vi "Controller LNLS Control PS Communication Loop.vi"(7 "Sync Objects":T1, 8 "error in (no error)":errorcluster, 11 "FOFB Configuration":T4={"FOFB Parameters"={"Network"={"FOFB Controller IP"="10.0.18.132", "LNLS Control Network IP"="10.0.18.132", "LNLS Control Network Power Supplies TCP Port"=4001, "LNLS Control Network FOFB Configuration TCP Port"=4002, "LNLS Control Network BPMs TCP Port"=4003, "Monitoring Data TCP Port"=3601, "Fast Archiver TCP Port"=3603, "Fast Command TCP Port"=3604, "TCP Listening Timeout"=-1}, "Fast Acquisition"={"Sampling Period"=320, "Data Buffer Size"=100, "Monitoring Period"=400000}, "Acquisition Network"=[{"Chassis Name"="BPM-Chassis01", "Variables"=[{"Variable Name"="AMP02AH", "Matrix Order"=2, "Plane"=enum."H", "On Correction"=TRUE}, {"Variable Name"="AMP02AV", "Matrix Order"=27, "Plane"=enum."V", "On Correction"=TRUE}, {"Variable Name"="AMP02BH", "Matrix Order"=3, "Plane"=enum."H", "On Correction"=TRUE}, {"Variable Name"="AMP02BV", "Matrix Order"=28, "Plane"=enum."V", "On Correction"=TRUE}, {"Variable Name"="AMP03AH", "Matrix Order"=4, "Plane"=enum."H", "On Correction"=TRUE}, {"Variable Name"="AMP03AV", "Matrix Order"=29, "Plane"=enum."V", "On Correction"=TRUE}, {"Variable Name"="AMP03BH", "Matrix Order"=5, "Plane"=enum."H", "On Correction"=TRUE}, {"Variable Name"="AMP03BV", "Matrix Order"=30, "Plane"=enum."V", "On Correction"=TRUE}, {"Variable Name"="AMP03CH", "Matrix Order"=6, "Plane"=enum."H", "On Correction"=FALSE}, {"Variable Name"="AMP03CV", "Matrix Order"=31, "Plane"=enum."V", "On Correction"=FALSE}]}, {"Chassis Name"="BPM-Chassis02", "Variables"=[{"Variable Name"="AMP04AH", "Matrix Order"=7, "Plane"=enum."H", "On Correction"=TRUE}, {"Variable Name"="AMP04AV", "Matrix Order"=32, "Plane"=enum."V", "On Correction"=TRUE}, {"Variable Name"="AMP04BH", "Matrix Order"=8, "Plane"=enum."H", "On Correction"=TRUE}, {"Variable Name"="AMP04BV", "Matrix Order"=33, "Plane"=enum."V", "On Correction"=TRUE}, {"Variable Name"="AMP05AH", "Matrix Order"=9, "Plane"=enum."H", "On Correction"=TRUE}, {"Variable Name"="AMP05AV", "Matrix Order"=34, "Plane"=enum."V", "On Correction"=TRUE}, {"Variable Name"="AMP05BH", "Matrix Order"=10, "Plane"=enum."H", "On Correction"=TRUE}, {"Variable Name"="AMP05BV", "Matrix Order"=35, "Plane"=enum."V", "On Correction"=TRUE}]}, {"Chassis Name"="BPM-Chassis03", "Variables"=[{"Variable Name"="AMP06AH", "Matrix Order"=11, "Plane"=enum."H", "On Correction"=TRUE}, {"Variable Name"="AMP06AV", "Matrix Order"=36, "Plane"=enum."V", "On Correction"=TRUE}, {"Variable Name"="AMP06BH", "Matrix Order"=12, "Plane"=enum."H", "On Correction"=TRUE}, {"Variable Name"="AMP06BV", "Matrix Order"=37, "Plane"=enum."V", "On Correction"=TRUE}, {"Variable Name"="AMP07AH", "Matrix Order"=13, "Plane"=enum."H", "On Correction"=TRUE}, {"Variable Name"="AMP07AV", "Matrix Order"=38, "Plane"=enum."V", "On Correction"=TRUE}, {"Variable Name"="AMP07BH", "Matrix Order"=14, "Plane"=enum."H", "On Correction"=TRUE}, {"Variable Name"="AMP07BV", "Matrix Order"=39, "Plane"=enum."V", "On Correction"=TRUE}]}, {"Chassis Name"="BPM-Chassis04", "Variables"=[{"Variable Name"="AMP08AH", "Matrix Order"=15, "Plane"=enum."H", "On Correction"=TRUE}, {"Variable Name"="AMP08AV", "Matrix Order"=40, "Plane"=enum."V", "On Correction"=TRUE}, {"Variable Name"="AMP08BH", "Matrix Order"=16, "Plane"=enum."H", "On Correction"=TRUE}, {"Variable Name"="AMP08BV", "Matrix Order"=41, "Plane"=enum."V", "On Correction"=TRUE}, {"Variable Name"="AMP09AH", "Matrix Order"=17, "Plane"=enum."H", "On Correction"=TRUE}, {"Variable Name"="AMP09AV", "Matrix Order"=42, "Plane"=enum."V", "On Correction"=TRUE}, {"Variable Name"="AMP09BH", "Matrix Order"=18, "Plane"=enum."H", "On Correction"=TRUE}, {"Variable Name"="AMP09BV", "Matrix Order"=43, "Plane"=enum."V", "On Correction"=TRUE}]}, {"Chassis Name"="BPM-Chassis05", "Variables"=[{"Variable Name"="AMP10AH", "Matrix Order"=19, "Plane"=enum."H", "On Correction"=TRUE}, {"Variable Name"="AMP10AV", "Matrix Order"=44, "Plane"=enum."V", "On Correction"=TRUE}, {"Variable Name"="AMP10BH", "Matrix Order"=20, "Plane"=enum."H", "On Correction"=TRUE}, {"Variable Name"="AMP10BV", "Matrix Order"=45, "Plane"=enum."V", "On Correction"=TRUE}, {"Variable Name"="AMU11AH", "Matrix Order"=21, "Plane"=enum."H", "On Correction"=TRUE}, {"Variable Name"="AMU11AV", "Matrix Order"=46, "Plane"=enum."V", "On Correction"=TRUE}, {"Variable Name"="AMU11BH", "Matrix Order"=22, "Plane"=enum."H", "On Correction"=TRUE}, {"Variable Name"="AMU11BV", "Matrix Order"=47, "Plane"=enum."V", "On Correction"=TRUE}]}, {"Chassis Name"="BPM-Chassis06", "Variables"=[{"Variable Name"="AMP12AH", "Matrix Order"=23, "Plane"=enum."H", "On Correction"=TRUE}, {"Variable Name"="AMP12AV", "Matrix Order"=48, "Plane"=enum."V", "On Correction"=TRUE}, {"Variable Name"="AMP12BH", "Matrix Order"=24, "Plane"=enum."H", "On Correction"=TRUE}, {"Variable Name"="AMP12BV", "Matrix Order"=49, "Plane"=enum."V", "On Correction"=TRUE}, {"Variable Name"="AMP01AH", "Matrix Order"=25, "Plane"=enum."H", "On Correction"=TRUE}, {"Variable Name"="AMP01AV", "Matrix Order"=50, "Plane"=enum."V", "On Correction"=TRUE}, {"Variable Name"="AMP01BH", "Matrix Order"=1, "Plane"=enum."H", "On Correction"=TRUE}, {"Variable Name"="AMP01BV", "Matrix Order"=26, "Plane"=enum."V", "On Correction"=TRUE}]}], "Actuation Network"=[{"Chassis Name"="PS-RA01B", "Variables"=[{"Variable Name"="ACH01B", "Matrix Order"=1, "Plane"=enum."H", "On Correction"=TRUE}, {"Variable Name"="ACV01B", "Matrix Order"=19, "Plane"=enum."V", "On Correction"=TRUE}, {"Variable Name"="ACH03A", "Matrix Order"=3, "Plane"=enum."H", "On Correction"=TRUE}, {"Variable Name"="ACV03A", "Matrix Order"=22, "Plane"=enum."V", "On Correction"=TRUE}, {"Variable Name"="ALV02A", "Matrix Order"=20, "Plane"=enum."V", "On Correction"=TRUE}, {"Variable Name"="ALV02B", "Matrix Order"=21, "Plane"=enum."V", "On Correction"=TRUE}, {"Variable Name"="ACH02", "Matrix Order"=2, "Plane"=enum."H", "On Correction"=TRUE}]}, {"Chassis Name"="PS-RA02B", "Variables"=[{"Variable Name"="ACH03B", "Matrix Order"=4, "Plane"=enum."H", "On Correction"=TRUE}, {"Variable Name"="ACV03B", "Matrix Order"=23, "Plane"=enum."V", "On Correction"=TRUE}, {"Variable Name"="ACH05A", "Matrix Order"=6, "Plane"=enum."H", "On Correction"=TRUE}, {"Variable Name"="ACV05A", "Matrix Order"=26, "Plane"=enum."V", "On Correction"=TRUE}, {"Variable Name"="ALV04A", "Matrix Order"=24, "Plane"=enum."V", "On Correction"=TRUE}, {"Variable Name"="ALV04B", "Matrix Order"=25, "Plane"=enum."V", "On Correction"=TRUE}, {"Variable Name"="ACH04", "Matrix Order"=5, "Plane"=enum."H", "On Correction"=TRUE}]}, {"Chassis Name"="PS-RA03B", "Variables"=[{"Variable Name"="ACH05B", "Matrix Order"=7, "Plane"=enum."H", "On Correction"=TRUE}, {"Variable Name"="ACV05B", "Matrix Order"=27, "Plane"=enum."V", "On Correction"=TRUE}, {"Variable Name"="ACH07A", "Matrix Order"=9, "Plane"=enum."H", "On Correction"=TRUE}, {"Variable Name"="ACV07A", "Matrix Order"=30, "Plane"=enum."V", "On Correction"=TRUE}, {"Variable Name"="ALV06A", "Matrix Order"=28, "Plane"=enum."V", "On Correction"=TRUE}, {"Variable Name"="ALV06B", "Matrix Order"=29, "Plane"=enum."V", "On Correction"=TRUE}, {"Variable Name"="ACH06", "Matrix Order"=8, "Plane"=enum."H", "On Correction"=TRUE}]}, {"Chassis Name"="PS-RA04B", "Variables"=[{"Variable Name"="ACH07B", "Matrix Order"=10, "Plane"=enum."H", "On Correction"=TRUE}, {"Variable Name"="ACV07B", "Matrix Order"=31, "Plane"=enum."V", "On Correction"=TRUE}, {"Variable Name"="ACH09A", "Matrix Order"=12, "Plane"=enum."H", "On Correction"=TRUE}, {"Variable Name"="ACV09A", "Matrix Order"=34, "Plane"=enum."V", "On Correction"=TRUE}, {"Variable Name"="ALV08A", "Matrix Order"=32, "Plane"=enum."V", "On Correction"=TRUE}, {"Variable Name"="ALV08B", "Matrix Order"=33, "Plane"=enum."V", "On Correction"=TRUE}, {"Variable Name"="ACH08", "Matrix Order"=11, "Plane"=enum."H", "On Correction"=TRUE}]}, {"Chassis Name"="PS-RA05B", "Variables"=[{"Variable Name"="ACH09B", "Matrix Order"=13, "Plane"=enum."H", "On Correction"=TRUE}, {"Variable Name"="ACV09B", "Matrix Order"=35, "Plane"=enum."V", "On Correction"=TRUE}, {"Variable Name"="ACH11A", "Matrix Order"=15, "Plane"=enum."H", "On Correction"=TRUE}, {"Variable Name"="ACV11A", "Matrix Order"=38, "Plane"=enum."V", "On Correction"=TRUE}, {"Variable Name"="ALV10A", "Matrix Order"=36, "Plane"=enum."V", "On Correction"=TRUE}, {"Variable Name"="ALV10B", "Matrix Order"=37, "Plane"=enum."V", "On Correction"=TRUE}, {"Variable Name"="ACH10", "Matrix Order"=14, "Plane"=enum."H", "On Correction"=TRUE}]}, {"Chassis Name"="PS-RA06B", "Variables"=[{"Variable Name"="ACH11B", "Matrix Order"=16, "Plane"=enum."H", "On Correction"=TRUE}, {"Variable Name"="ACV11B", "Matrix Order"=39, "Plane"=enum."V", "On Correction"=TRUE}, {"Variable Name"="ACH01A", "Matrix Order"=18, "Plane"=enum."H", "On Correction"=TRUE}, {"Variable Name"="ACV01A", "Matrix Order"=42, "Plane"=enum."V", "On Correction"=TRUE}, {"Variable Name"="ALV12A", "Matrix Order"=40, "Plane"=enum."V", "On Correction"=TRUE}, {"Variable Name"="ALV12B", "Matrix Order"=41, "Plane"=enum."V", "On Correction"=TRUE}, {"Variable Name"="ACH12", "Matrix Order"=17, "Plane"=enum."H", "On Correction"=TRUE}]}]}, "Number of Acquisition Chassis"=6, "Number of Actuation Chassis"=6, "Number of BPM Readings"=50, "BPM Reading Names"=["AMP01BH", "AMP02AH", "AMP02BH", "AMP03AH", "AMP03BH", "AMP03CH", "AMP04AH", "AMP04BH", "AMP05AH", "AMP05BH", "AMP06AH", "AMP06BH", "AMP07AH", "AMP07BH", "AMP08AH", "AMP08BH", "AMP09AH", "AMP09BH", "AMP10AH", "AMP10BH", "AMU11AH", "AMU11BH", "AMP12AH", "AMP12BH", "AMP01AH", "AMP01BV", "AMP02AV", "AMP02BV", "AMP03AV", "AMP03BV", "AMP03CV", "AMP04AV", "AMP04BV", "AMP05AV", "AMP05BV", "AMP06AV", "AMP06BV", "AMP07AV", "AMP07BV", "AMP08AV", "AMP08BV", "AMP09AV", "AMP09BV", "AMP10AV", "AMP10BV", "AMU11AV", "AMU11BV", "AMP12AV", "AMP12BV", "AMP01AV"], "Selected BPM Readings"=[0, 1, 2, 3, 4, 6, 7, 8, 9, 10, 11, 12, 13, 14, 15, 16, 17, 18, 19, 20, 21, 22, 23, 24, 25, 26, 27, 28, 29, 31, 32, 33, 34, 35, 36, 37, 38, 39, 40, 41, 42, 43, 44, 45, 46, 47, 48, 49], "Number of Correctors"=42, "Corrector Names"=["ACH01B", "ACH02", "ACH03A", "ACH03B", "ACH04", "ACH05A", "ACH05B", "ACH06", "ACH07A", "ACH07B", "ACH08", "ACH09A", "ACH09B", "ACH10", "ACH11A", "ACH11B", "ACH12", "ACH01A", "ACV01B", "ALV02A", "ALV02B", "ACV03A", "ACV03B", "ALV04A", "ALV04B", "ACV05A", "ACV05B", "ALV06A", "ALV06B", "ACV07A", "ACV07B", "ALV08A", "ALV08B", "ACV09A", "ACV09B", "ALV10A", "ALV10B", "ACV11A", "ACV11B", "ALV12A", "ALV12B", "ACV01A"], "Selected Correctors"=[0, 1, 2, 3, 4, 5, 6, 7, 8, 9, 10, 11, 12, 13, 14, 15, 16, 17, 18, 19, 20, 21, 22, 23, 24, 25, 26, 27, 28, 29, 30, 31, 32, 33, 34, 35, 36, 37, 38, 39, 40, 41], "Response Matrix"=[[[-1.09330819, 0.83238826, -1.93923182, -0.39618552, -0.98307235, -1.88049663, 1.00296681, -0.19883275, -1.65005616, -0.55712353, 0.68544531, -0.70274756, -0.65496658, 0.05515979, -0.38935, 0.30350319, -0.13918837, -0.00011801, -0.21517587, -0.53815631, 0.44595451, 0.75898104, -0.44725813, -1.09971674, -0.46972415, -0.36841134, -0.07750092, 0.48295386, 0.47744403, 2.130847, 0.4681161, 0.39999255, -0.15570575, 0.89687682, 0.94383742, 1.1290593, -0.75786475, 0.54152616, 0.43217361, 0.98547068, 0.07993329, 0.29159442, 0.45045343, 0.73064824, 0.57741329, 0.86763439, 1.47745915, 1.05383194, 0.75658237, 0.2512502]]], "Reference Orbit"=array50x42[2100 elements], "Correction Matrix"=array1x42x48[2016 elements], "FPGA Filter Sets"=[], "Acquisition Chassis Names"=["PS-RA01B", "PS-RA02B", "PS-RA03B", "PS-RA04B", "PS-RA05B", "PS-RA06B"], "Actuation Chassis Names"=[], "Acquisition Variables"=[{"Variable Name"="ACH01B", "Chassis Name"="PS-RA01B"}, {"Variable Name"="ACH02", "Chassis Name"="PS-RA01B"}, {"Variable Name"="ACH03A", "Chassis Name"="PS-RA01B"}, {"Variable Name"="ACH03B", "Chassis Name"="PS-RA02B"}, {"Variable Name"="ACH04", "Chassis Name"="PS-RA02B"}, {"Variable Name"="ACH05A", "Chassis Name"="PS-RA02B"}, {"Variable Name"="ACH05B", "Chassis Name"="PS-RA03B"}, {"Variable Name"="ACH06", "Chassis Name"="PS-RA03B"}, {"Variable Name"="ACH07A", "Chassis Name"="PS-RA03B"}, {"Variable Name"="ACH07B", "Chassis Name"="PS-RA04B"}, {"Variable Name"="ACH08", "Chassis Name"="PS-RA04B"}, {"Variable Name"="ACH09A", "Chassis Name"="PS-RA04B"}, {"Variable Name"="ACH09B", "Chassis Name"="PS-RA05B"}, {"Variable Name"="ACH10", "Chassis Name"="PS-RA05B"}, {"Variable Name"="ACH11A", "Chassis Name"="PS-RA05B"}, {"Variable Name"="ACH11B", "Chassis Name"="PS-RA06B"}, {"Variable Name"="ACH12", "Chassis Name"="PS-RA06B"}, {"Variable Name"="ACH01A", "Chassis Name"="PS-RA06B"}, {"Variable Name"="ACV01B", "Chassis Name"="PS-RA01B"}, {"Variable Name"="ALV02A", "Chassis Name"="PS-RA01B"}, {"Variable Name"="ALV02B", "Chassis Name"="PS-RA01B"}, {"Variable Name"="ACV03A", "Chassis Name"="PS-RA01B"}, {"Variable Name"="ACV03B", "Chassis Name"="PS-RA02B"}, {"Variable Name"="ALV04A", "Chassis Name"="PS-RA02B"}, {"Variable Name"="ALV04B", "Chassis Name"="PS-RA02B"}, {"Variable Name"="ACV05A", "Chassis Name"="PS-RA02B"}, {"Variable Name"="ACV05B", "Chassis Name"="PS-RA03B"}, {"Variable Name"="ALV06A", "Chassis Name"="PS-RA03B"}, {"Variable Name"="ALV06B", "Chassis Name"="PS-RA03B"}, {"Variable Name"="ACV07A", "Chassis Name"="PS-RA03B"}, {"Variable Name"="ACV07B", "Chassis Name"="PS-RA04B"}, {"Variable Name"="ALV08A", "Chassis Name"="PS-RA04B"}, {"Variable Name"="ALV08B", "Chassis Name"="PS-RA04B"}, {"Variable Name"="ACV09A", "Chassis Name"="PS-RA04B"}, {"Variable Name"="ACV09B", "Chassis Name"="PS-RA05B"}, {"Variable Name"="ALV10A", "Chassis Name"="PS-RA05B"}, {"Variable Name"="ALV10B", "Chassis Name"="PS-RA05B"}, {"Variable Name"="ACV11A", "Chassis Name"="PS-RA05B"}, {"Variable Name"="ACV11B", "Chassis Name"="PS-RA06B"}, {"Variable Name"="ALV12A", "Chassis Name"="PS-RA06B"}, {"Variable Name"="ALV12B", "Chassis Name"="PS-RA06B"}, {"Variable Name"="ACV01A", "Chassis Name"="PS-RA06B"}], "Actuation Variables"=[{"Variable Name"="", "Chassis Name"=""}, {"Variable Name"="", "Chassis Name"=""}, {"Variable Name"="", "Chassis Name"=""}, {"Variable Name"="", "Chassis Name"=""}, {"Variable Name"="", "Chassis Name"=""}, {"Variable Name"="", "Chassis Name"=""}], "PS Matrix Mapping"=[], "Inverse PS Matrix Mapping"=[], "BPM Matrix Mapping"=[], "Inverse BPM Matrix Mapping"=[[0, 0, 0, 0, 0, 0, 16843008, 16843009, 16843009, 16843009, 16843009, 16843009, 257, 0, 516538096, 516549112, 95143185, 0, 0, 516547907, 33975304, 49, 516550840, 0, 0, 516513040, 2, 0, 0, 0, 0, 0, 516539392, 516544576, 95143185, 0, 0, 516553163, 33975304, 49, 516550840, 0, 0, 516513112, 2, 0, 0, 0, 0, 0]], "BPM Planes"=[enum."H", enum."H", enum."H", enum."H", enum."H", enum."H", enum."H", enum."H", enum."H", enum."H", enum."H", enum."H", enum."H", enum."H", enum."H", enum."H", enum."H", enum."H", enum."V", enum."V", enum."V", enum."V", enum."V", enum."V", enum."V", enum."V", enum."V", enum."V", enum."V", enum."V", enum."V", enum."V", enum."V", enum."V", enum."V", enum."V", enum."V", enum."V", enum."V", enum."V", enum."V", enum."V"], "Corrector Planes"=[]}) -> (0 "error out":errorcluster)   [LabVIEW 2011, in "Controller VIs.lvlib"]
uses:
  Controller VIs.lvlib
  Types Definitions/Type FOFB Configuration.ctl
  Types Definitions/Type FOFB Parameters.ctl
  Types Definitions/Type Network Configuration.ctl
  Types Definitions/Type FA Configuration.ctl
  Types Definitions/Type Acquisition Network Configuration.ctl
  Types Definitions/Type Actuation Network Configuration.ctl
  Types Definitions/Type Synchronization Objects.ctl
  Types Definitions/Type Blocking Synchronization Objects.ctl
  Types Definitions/Type Monitoring Data.ctl
  Types Definitions/Type Operation Mode State.ctl
  Types Definitions/Type Diagnostics Data.ctl
  Types Definitions/Type CPU Loads Array.ctl
  Types Definitions/Type CPU Loads.ctl
  Types Definitions/Type Non-blocking Synchronization Objects.ctl
  Types Definitions/Type FOFB Variables.ctl
  Types Definitions/Type Actuation State.ctl
  Types Definitions/Type TCP State.ctl
  <vilib>/Platform/TimedLoop/XDataNode/timing_clust.ctl
  <vilib>/Platform/TimedLoop/XDataNode/nitl_modes.ctl
  <vilib>/Platform/TimedLoop/XDataNode/wakeup.ctl
  Controller Global Variables/Monitoring Data.vi
  LNLS Control VIs/LNLS Control Saturation minus10 10.vi
  <vilib>/Platform/TimedLoop/XDataNode/XDataNode.xnode
  LNLS Control VIs.lvlib
  Common VIs.lvlib
  Misc VIs.lvlib
  Controller Global Variables.lvlib
  <vilib>/Platform/TimedLoop/XDataNode/XDNodeRunTimeDep.lvlib
  Type Definitions.lvlib
panel:
  in  "send":bool
  in  "PS Status (On correction?)":bool[](array[boolean])=[TRUE, TRUE, TRUE, TRUE, TRUE, TRUE, TRUE, TRUE, TRUE, TRUE, TRUE, TRUE, TRUE, TRUE, TRUE, TRUE, TRUE, TRUE, TRUE, TRUE, TRUE, TRUE, TRUE, TRUE, TRUE, TRUE, TRUE, TRUE, TRUE, TRUE, TRUE, TRUE, TRUE, TRUE, TRUE, TRUE, TRUE, TRUE, TRUE, TRUE, TRUE, TRUE]
  in  "PS Status (ON/OFF)":bool[](array[boolean])=[TRUE, TRUE, TRUE, TRUE, TRUE, TRUE, TRUE, TRUE, TRUE, TRUE, TRUE, TRUE, TRUE, TRUE, TRUE, TRUE, TRUE, TRUE, TRUE, TRUE, TRUE, TRUE, TRUE, TRUE, TRUE, TRUE, TRUE, TRUE, TRUE, TRUE, TRUE, TRUE, TRUE, TRUE, TRUE, TRUE, TRUE, TRUE, TRUE, TRUE, TRUE, TRUE]
  in  "PS Setpoints":dbl[](array[numeric])=[0.0, 0.0, 0.0, 0.0, 0.0, 0.0, 0.0, 0.0, 0.0, 0.0, 0.0, 0.0, 0.0, 0.0, 0.0, 0.0, 0.0, 0.0, 0.0, 0.0, 0.0, 0.0, 0.0, 0.0, 0.0, 0.0, 0.0, 0.0, 0.0, 0.0, 0.0, 0.0, 0.0, 0.0, 0.0, 0.0, 0.0, 0.0, 0.0, 0.0, 0.0, 0.0]
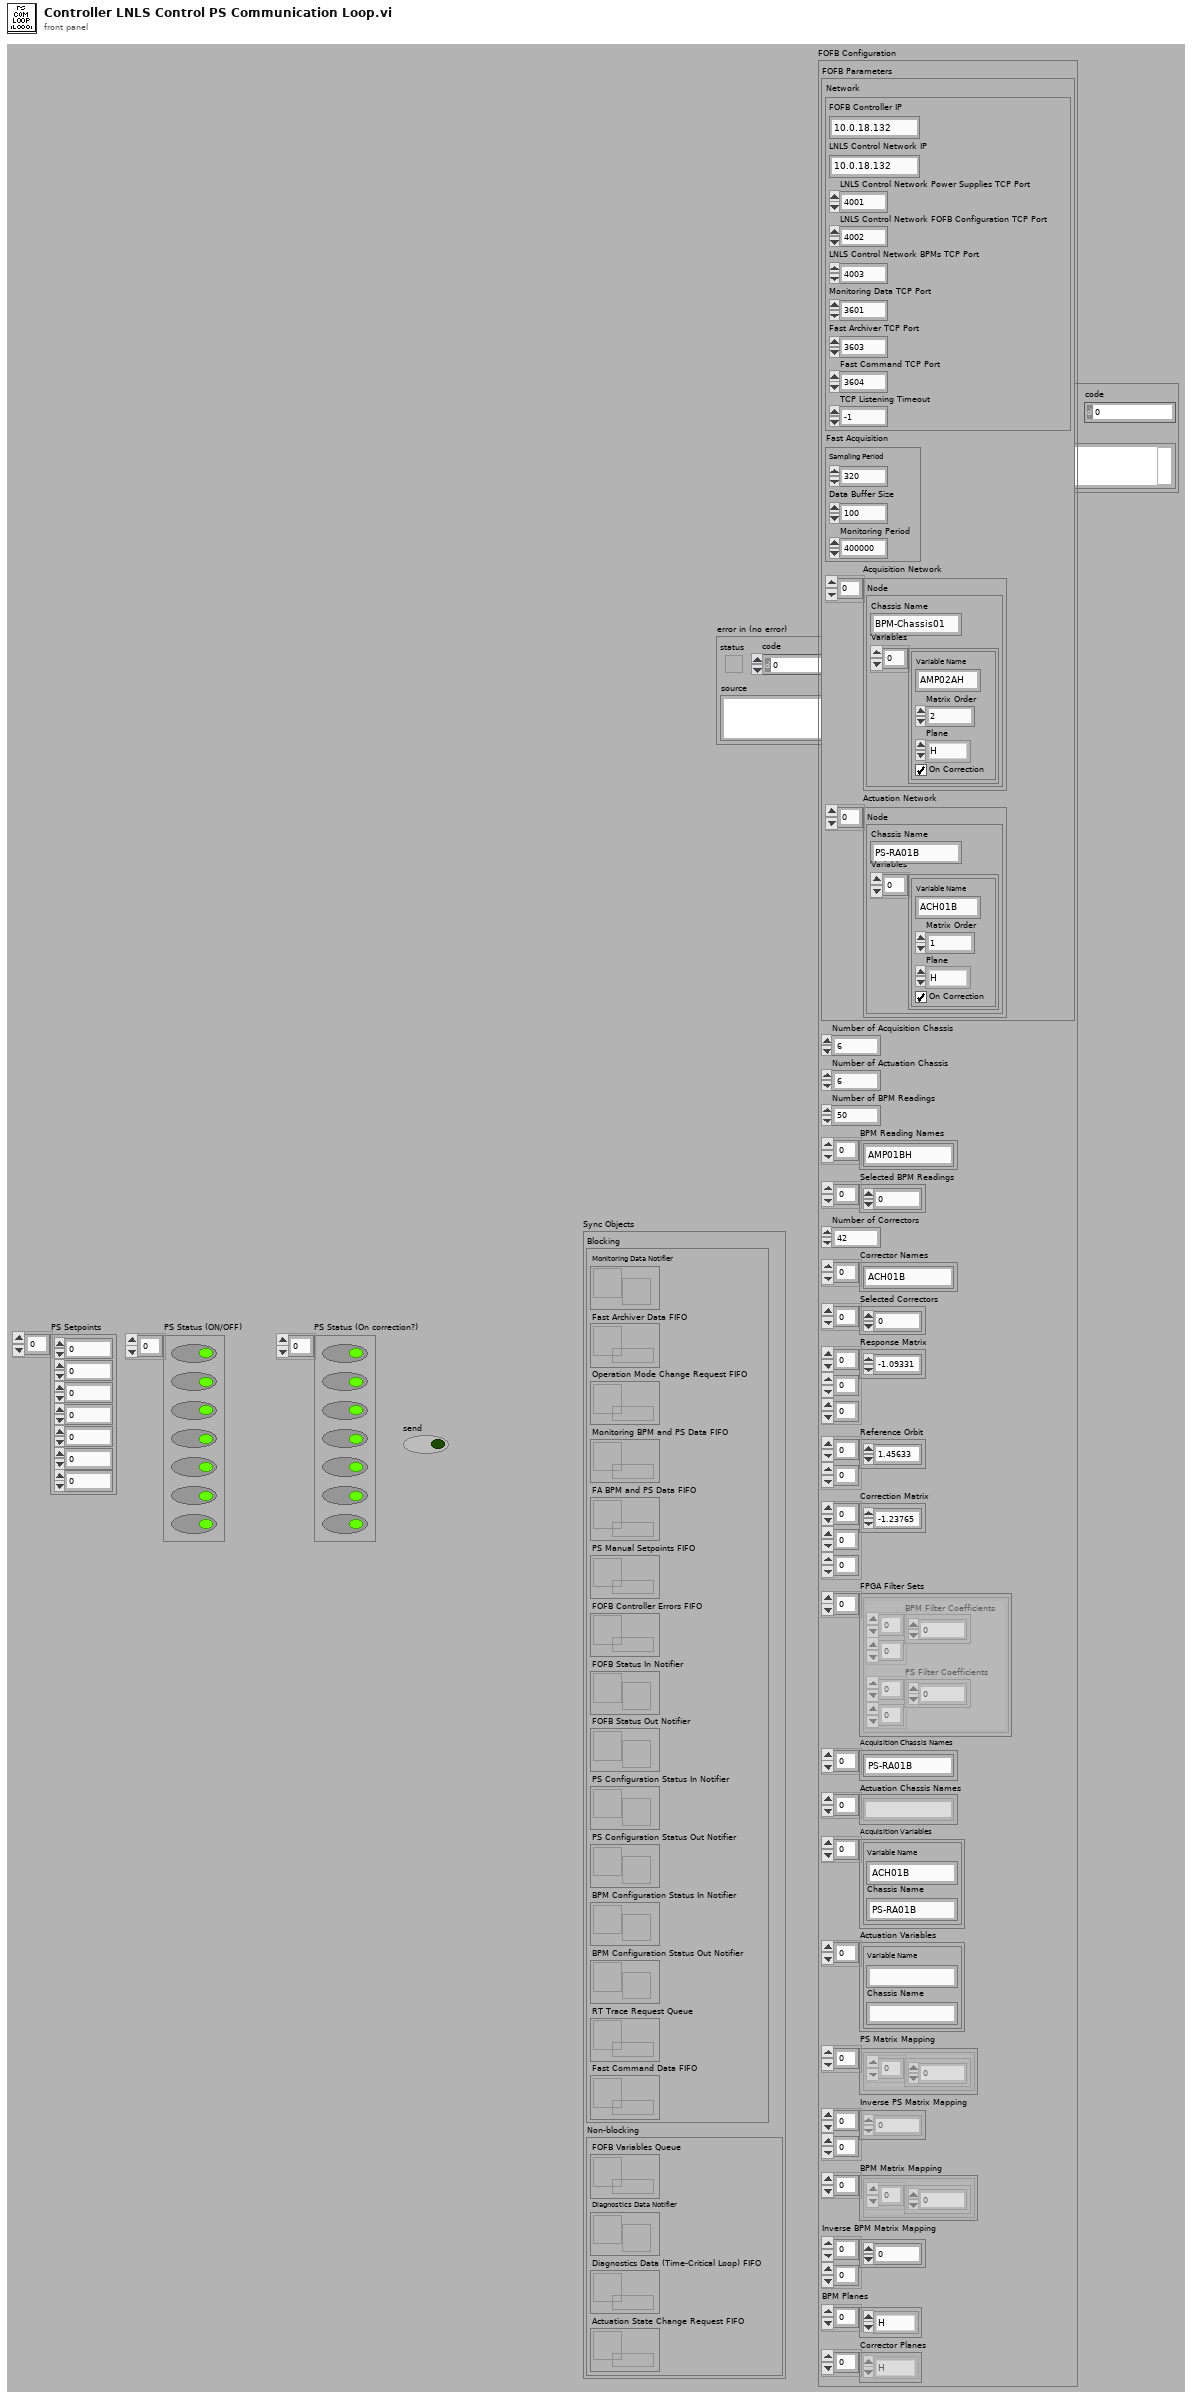
[diagram p1: front panel]
types:
  T1 = typedef "Type Definitions.lvlib/Type Synchronization Objects.ctl" = cluster{"Blocking":T2, "Non-blocking":T3}
  T2 = typedef "Type Definitions.lvlib/Type Blocking Synchronization Objects.ctl" = cluster{"Monitoring Data Notifier":refnum<notifier>, "Fast Archiver Data FIFO":refnum<queue>, "Operation Mode Change Request FIFO":refnum<k33>, "Monitoring BPM and PS Data FIFO":refnum<k33>, "FA BPM and PS Data FIFO":refnum<k33>, "PS Manual Setpoints FIFO":refnum<k33>, "FOFB Controller Errors FIFO ":refnum<k33>, "FOFB Status In Notifier":refnum<notifier>, "FOFB Status Out Notifier":refnum<notifier>, "PS Configuration Status In Notifier":refnum<notifier>, "PS Configuration Status Out Notifier":refnum<notifier>, "BPM Configuration Status In Notifier":refnum<notifier>, "BPM Configuration Status Out Notifier":refnum<notifier>, "RT Trace Request Queue":refnum<queue>, "Fast Command Data FIFO":refnum<k33>}
  T3 = typedef "Type Definitions.lvlib/Type Non-blocking Synchronization Objects.ctl" = cluster{"FOFB Variables Queue":refnum<queue>, "Diagnostics Data Notifier":refnum<notifier>, "Diagnostics Data (Time-Critical Loop) FIFO":refnum<k33>, "Actuation State Change Request FIFO":refnum<k33>}
  T4 = typedef "Type Definitions.lvlib/Type FOFB Configuration.ctl" = cluster{"FOFB Parameters":T5, "Number of Acquisition Chassis":i32, "Number of Actuation Chassis":i32, "Number of BPM Readings":i32, "BPM Reading Names":string[], "Selected BPM Readings":u32[], "Number of Correctors":i32, "Corrector Names":string[], "Selected Correctors":u32[], "Response Matrix":dbl[][][], "Reference Orbit":dbl[][], "Correction Matrix":dbl[][][], "FPGA Filter Sets":cluster{"BPM Filter Coefficients":dbl[][], "PS Filter Coefficients":dbl[][]}[], "Acquisition Chassis Names":string[], "Actuation Chassis Names":string[], "Acquisition Variables":cluster{"Variable Name":string, "Chassis Name":string}[], "Actuation Variables":cluster{"Variable Name":string, "Chassis Name":string}[], "PS Matrix Mapping":cluster{u32[]}[], "Inverse PS Matrix Mapping":u32[][], "BPM Matrix Mapping":cluster{u32[]}[], "Inverse BPM Matrix Mapping":u32[][], "BPM Planes":enum8{"H", "V"}[], "Corrector Planes":enum8{"H", "V"}[]}
  T5 = typedef "Type Definitions.lvlib/Type FOFB Parameters.ctl" = cluster{"Network":T6, "Fast Acquisition":T7, "Acquisition Network":T8, "Actuation Network":T9}
  T6 = typedef "Type Definitions.lvlib/Type Network Configuration.ctl" = cluster{"FOFB Controller IP":string, "LNLS Control Network IP":string, "LNLS Control Network Power Supplies TCP Port":u16, "LNLS Control Network FOFB Configuration TCP Port":u16, "LNLS Control Network BPMs TCP Port":u16, "Monitoring Data TCP Port":u16, "Fast Archiver TCP Port":u16, "Fast Command TCP Port":u16, "TCP Listening Timeout":i32}
  T7 = typedef "Type Definitions.lvlib/Type FA Configuration.ctl" = cluster{"Sampling Period":u32, "Data Buffer Size":u32, "Monitoring Period":u32}
  T8 = typedef "Type Definitions.lvlib/Type Acquisition Network Configuration.ctl" = cluster{"Chassis Name":string, "Variables":cluster{"Variable Name":string, "Matrix Order":u32, "Plane":enum8{"H", "V"}, "On Correction":bool}[]}[]
  T9 = typedef "Type Definitions.lvlib/Type Actuation Network Configuration.ctl" = cluster{"Chassis Name":string, "Variables":cluster{"Variable Name":string, "Matrix Order":u32, "Plane":enum8{"H", "V"}, "On Correction":bool}[]}[]
  T10 = typedef "Type Definitions.lvlib/Type TCP State.ctl" = enum16{"Idle", "Wait Connection", "Read Data", "Process Data", "Write Data", "Close Connection"}
  T11 = typedef "XDNodeRunTimeDep.lvlib/timing_clust.ctl" = cluster{"Expected End [f-1]":u64, "Actual End [f-1]":u64, "Finished Late? [f-1]":bool, "Expected End [i-1]":u64, "Actual End [i-1]":u64, "Finished Late? [i-1]":bool, "Expected Start [i]":u64, "Actual Start [i]":u64, "Expected Start [f]":u64, "Actual Start [f]":u64, "Source Name":string, "Structure Name":string, "Period":i64, "Deadline":i64, "Offset":i64, "Start":i64, "Priority":i32, "Timeout":i32, "Mode":T12, "Wakeup Reason":T13, "Error":errorcluster, "Source Type":string, "Secondary Source Type":string, "Global End Time":u64, "Global Start Time":u64, "Frame Duration":u64, "Iteration Duration":u64, "Assigned CPU":i32, "I/O Scan Engine Mode":u32}
  T12 = typedef "XDNodeRunTimeDep.lvlib/nitl_modes.ctl" = enum32{"No Change", "Process missed periods, maintain original phase", "Discard missed periods, maintain original phase", "Process missed periods, ignore original phase", "Discard missed periods, ignore original phase"}
  T13 = typedef "XDNodeRunTimeDep.lvlib/wakeup.ctl" = enum32{"Normal", "Aborted", "Asynchronous wakeup", "Timing source error", "Timed loop error", "Timeout"}
  T14 = typedef "Type Definitions.lvlib/Type Monitoring Data.ctl" = cluster{"Timestamp":timestamp, "BPM Readings":dbl[], "PS Readings":dbl[], "PS FOFB Setpoints":dbl[], "PS Status per Rack":u8[], "PS ON-OFF per Rack":u8[], "Operation Mode":T15, "Diagnostics Data":T16, "Controller Status Table":i32[]}
  T15 = typedef "Type Definitions.lvlib/Type Operation Mode State.ctl" = enum8{"Idle Mode", "Manual Mode", "FOFB Mode"}
  T16 = typedef "Type Definitions.lvlib/Type Diagnostics Data.ctl" = cluster{"Time-Critical Loop Missed Iterations":u32, "Time-Critical Loop Execution Time (usec)":u32, "Available Memory (bytes)":u32, "CPU Loads Array":T17}
  T17 = typedef "Type Definitions.lvlib/Type CPU Loads Array.ctl" = T18[]
  T18 = typedef "Type Definitions.lvlib/Type CPU Loads.ctl" = cluster{"Total (%)":dbl, "Time Critical (%)":dbl, "Timed Structures (%)":dbl, "High (%)":dbl, "Above Normal (%)":dbl, "Normal (%)":dbl, "Background (%)":dbl, "Idle (%)":dbl, "ISR (%)":dbl}
  T19 = typedef "Type Definitions.lvlib/Type LOCON_BIPOLAR_16BITS.ctl" = cluster{"priority":u8, "flags":u8, "analog value":u16, "status":u8}
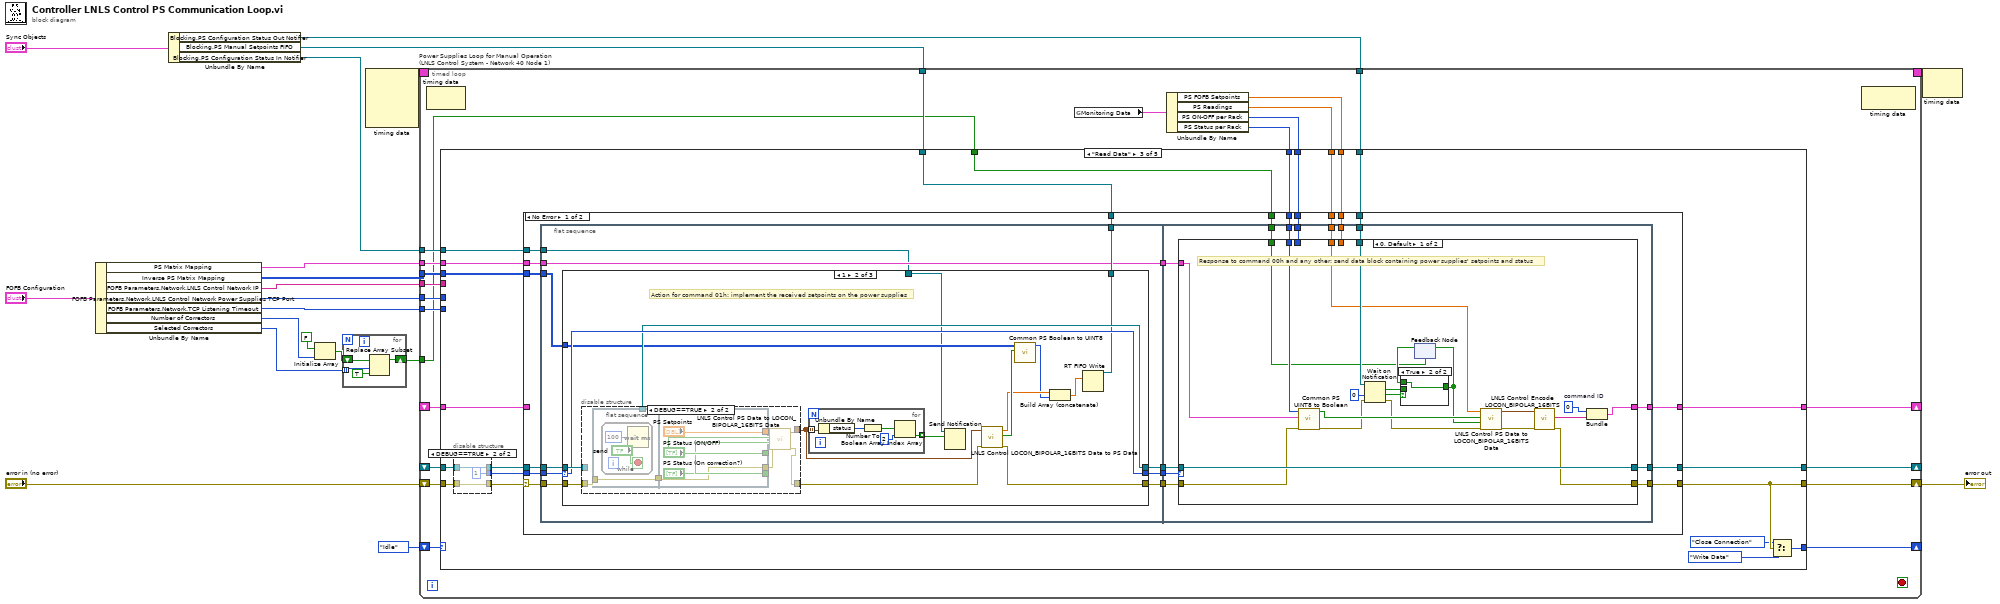
[diagram p0: block diagram]
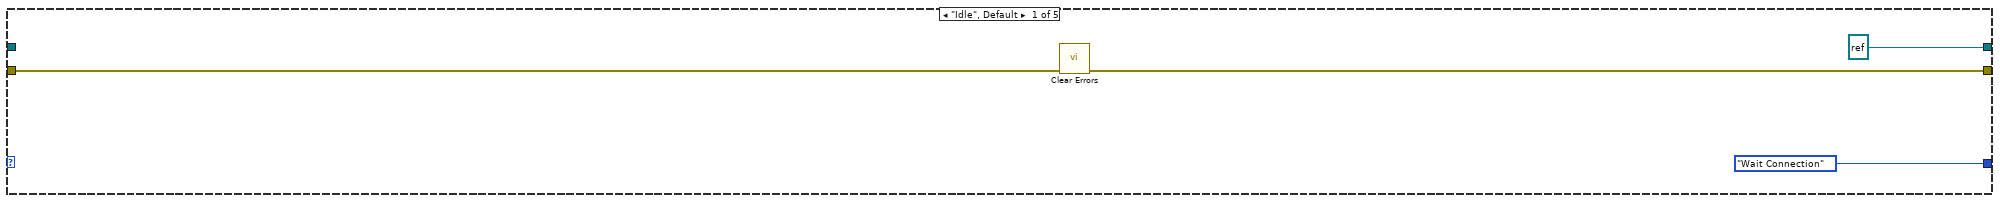
[diagram p2: hidden frame]
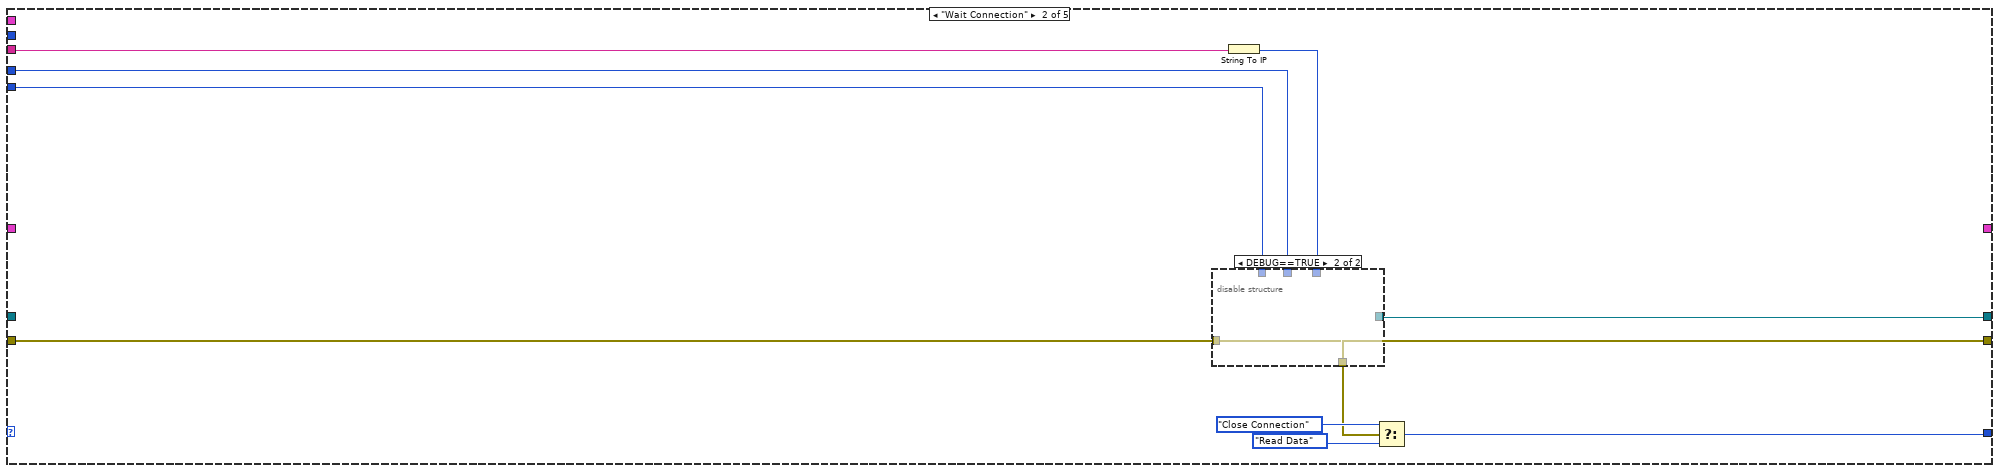
[diagram p3: hidden frame]
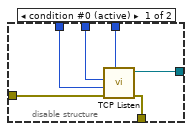
[diagram p4: hidden frame]
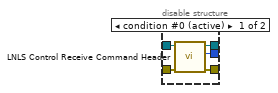
[diagram p5: hidden frame]
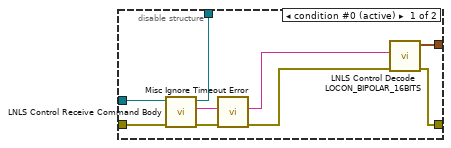
[diagram p7: hidden frame]
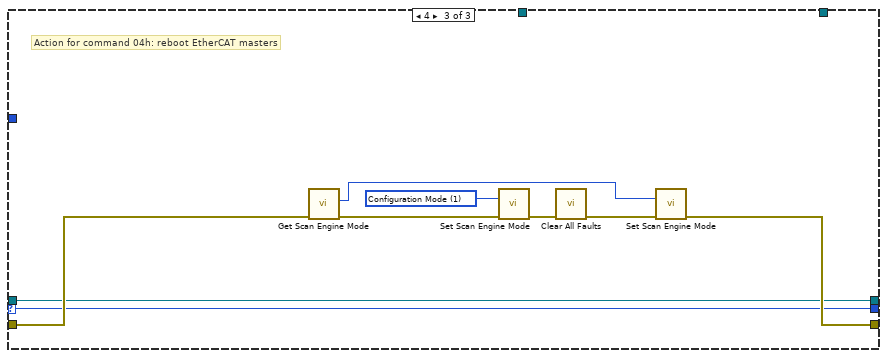
[diagram p8: hidden frame]
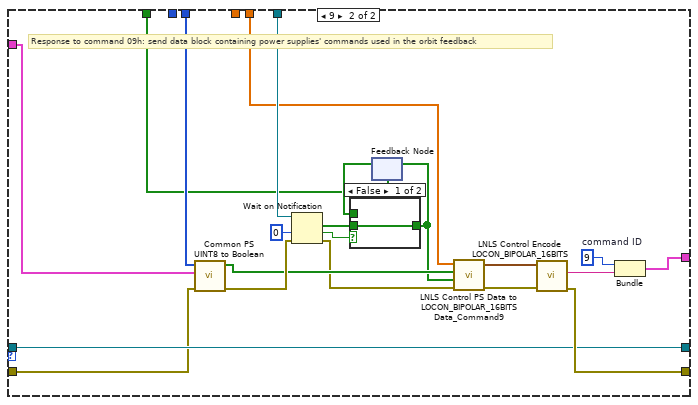
[diagram p10: hidden frame]
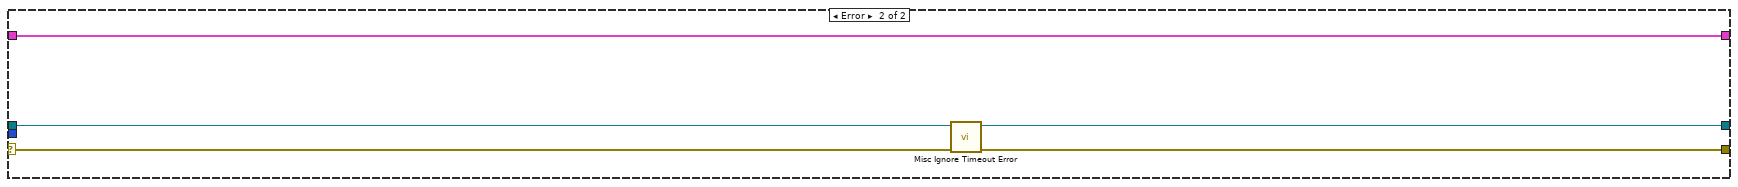
[diagram p12: hidden frame]
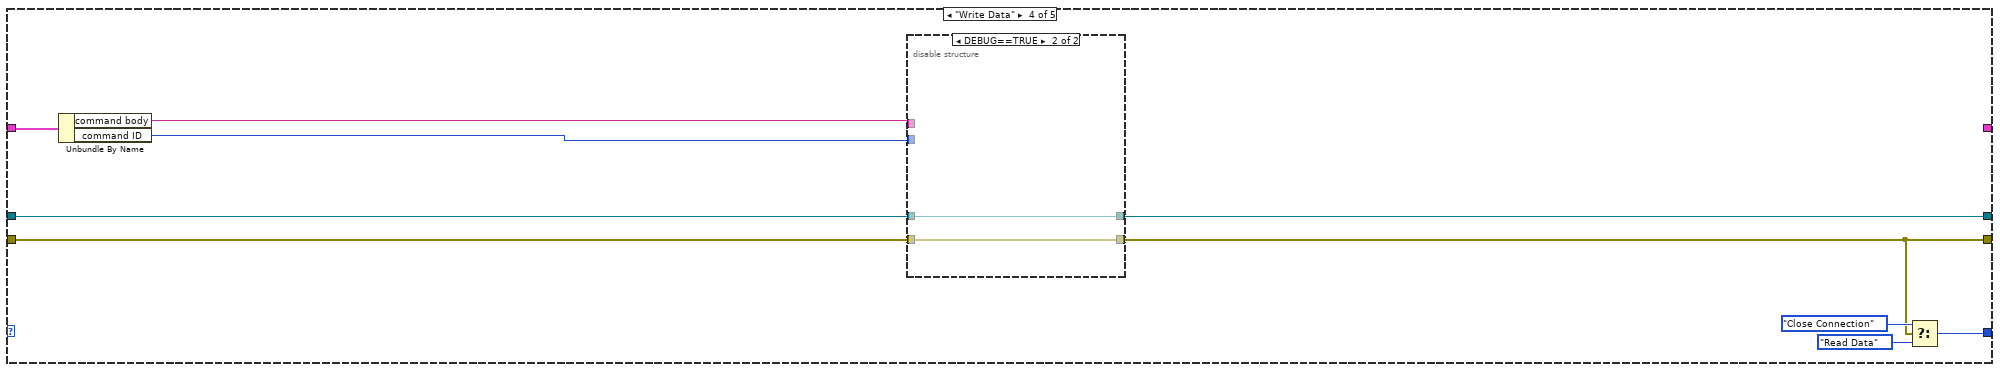
[diagram p13: hidden frame]
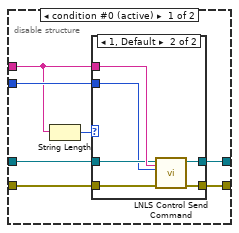
[diagram p14: hidden frame]
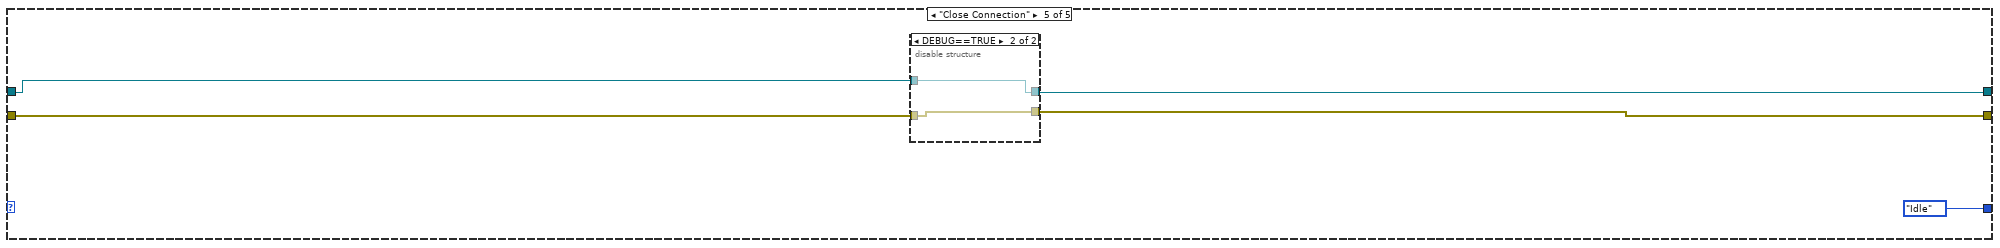
[diagram p16: hidden frame]
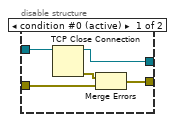
[diagram p17: hidden frame]
diagram:
  n1 = Unbundle By Name("FOFB Configuration") -> ("PS Matrix Mapping"=w13:cluster{u32[]}[], "Inverse PS Matrix Mapping"=w14:u32[][], "FOFB Parameters.Network.LNLS Control Network IP"=w15:string, "FOFB Parameters.Network.LNLS Control Network Power Supplies TCP Port"=w12:u16, "FOFB Parameters.Network.TCP Listening Timeout"=w11:i32, "Number of Correctors"=w5:i32, "Selected Correctors"=w3:u32[])
  n2 = Unbundle By Name("Sync Objects") -> ("Blocking.PS Configuration Status Out Notifier"=w8:refnum<notifier>, "Blocking.PS Manual Setpoints FIFO"=w1:refnum<k33>, "Blocking.PS Configuration Status In Notifier"=w7:refnum<notifier>)
  n3 = Initialize Array(FALSE, w5) -> (w4:bool[])
  n4 = for {
    tunnel: w3 -> [w24] mode=indexing
    shift-right: [w21] -> w2
    shift-left: w4 -> [w23]
    n5 = Replace Array Subset(array=w23, new element=TRUE ("new element/subarray"), index=w24) -> (w21:bool[])
  }
  n6 = node-c288() -> (w10:T11)  [unwired: 4 in]
  n7 = timed-loop "Power Supplies Loop for Manual Operation (LNLS Control System - Network 40 Node 1)" {
    shift-right: [w44] -> _
    shift-left: Type_TCP_State."Idle" ("f") -> [w46]
    shift-right: [w45] -> _
    shift-left: _ -> [w43]
    shift-right: [w25] -> w18
    shift-left: "error in (no error)" -> [w39]
    shift-right: [w41] -> _
    shift-left: _ -> [w40]
    tunnel: w12 -> [w42]
    tunnel: w15 -> [w38]
    tunnel: w14 -> [w37]
    tunnel: w13 -> [w36]
    tunnel: w11 -> [w35]
    tunnel: w1 -> [w31]
    timing: w10 -> [_]
    timing-out: [_] -> w9
    tunnel: w8 -> [w28]
    tunnel: w7 -> [w27]
    tunnel: w2 -> [w26]
    stop <- _ stop-if-true
    n8 = node-c288() -> ()  [unwired: 1 in, 1 out]
    n9 = global read "Monitoring Data.vi" "Monitoring Data"() -> (w32:T14)
    n10 = Unbundle By Name(w32) -> ("PS FOFB Setpoints"=w34:dbl[], "PS Readings"=w33:dbl[], "PS ON-OFF per Rack"=w29:u8[], "PS Status per Rack"=w30:u8[])
    n11 = case shown="\"Read Data\"" w46 {
      tunnel: [refnum<k5> refnum ("connection ID") w59 w91 w251 w278] -> w45
      tunnel: [w50 w54 w89 w250 w275] -> w25
      tunnel: [Type_TCP_State."Wait Connection" w62 w90 w255 Type_TCP_State."Idle"] -> w44
      tunnel: w43 -> [_ _ w87 w253 w279]
      tunnel: w39 -> [w49 w55 w88 w252 w276]
      tunnel: w42 -> [_ w58 _ _ _]
      tunnel: [_ _ w84 _ _] -> w41
      tunnel: w40 -> [_ _ w82 w254 _]
      tunnel: w38 -> [_ w56 _ _ _]
      tunnel: w37 -> [_ _ w80 _ _]
      tunnel: w36 -> [_ _ w79 _ _]
      tunnel: w35 -> [_ w53 _ _ _]
      tunnel: w34 -> [_ _ w70 _ _]
      tunnel: w33 -> [_ _ w71 _ _]
      tunnel: w30 -> [_ _ w78 _ _]
      tunnel: w31 -> [_ _ w77 _ _]
      tunnel: w29 -> [_ _ w76 _ _]
      tunnel: w28 -> [_ _ w75 _ _]
      tunnel: w27 -> [_ _ w73 _ _]
      tunnel: w26 -> [_ _ w72 _ _]
      frame "Idle", Default {
        n12 = call <vilib>:"Clear Errors.vi"("error in (no error)"=w49) -> ("error out"=w50:errorcluster)  [unwired: 6 in]
      }
      frame "Wait Connection" {
        n13 = String To IP(1:w56) -> (0:w57:u32)
        n14 = disable-structure shown="DEBUG==TRUE" {
          disable-tunnel: [w68 _] -> w59
          disable-tunnel: w58 -> [w67 _]
          disable-tunnel: w57 -> [w66 _]
          disable-tunnel: w55 -> [w65 w69]
          disable-tunnel: [w64 w69] -> w54
          disable-tunnel: w53 -> [w63 _]
          frame condition #0 (active) {
            n15 = call <vilib>:"TCP Listen.vi"("net address"=w66, "error in (no error)"=w65, "timeout ms (wait forever: -1)"=w63, "port"=w67) -> ("error out"=w64:errorcluster, "connection ID"=w68:refnum<k5>)  [unwired: 3 in, 3 out]
          }
          frame condition #1 {
          }
        }
        n16 = Select(t=Type_TCP_State."Close Connection", s=w54, f=Type_TCP_State."Read Data") -> (s? t:f=w62:T10)
      }
      frame "Read Data" {
        n17 = disable-structure shown="DEBUG==TRUE" {
          disable-tunnel: w88 -> [w96 w99]
          disable-tunnel: w87 -> [w95 w98]
          disable-tunnel: [w94 w98] -> w86
          disable-tunnel: [w93 w99] -> w83
          disable-tunnel: [w92 u8 1 ("command ID")] -> w74
          frame condition #0 (active) {
            n18 = call "LNLS Control Receive Command Header.vi"("error in (no error)"=w96, "connection ID"=w95) -> ("error out"=w93:errorcluster, "command ID"=w92:u8, "connection ID out"=w94:refnum<k5>)  [unwired: 7 in]
          }
          frame condition #1 {
          }
        }
        n19 = case shown="No Error" w83 {
          selector: w83 -> [w114 w244]
          tunnel: [w119 w247] -> w91
          tunnel: [w118 w245] -> w89
          tunnel: w86 -> [w117 w247]
          tunnel: w74 -> [w116 _]
          tunnel: [w115 w246] -> w84
          tunnel: w82 -> [_ w246]
          tunnel: w80 -> [w110 _]
          tunnel: w79 -> [w108 _]
          tunnel: w70 -> [w107 _]
          tunnel: w71 -> [w106 _]
          tunnel: w78 -> [w105 _]
          tunnel: w77 -> [w104 _]
          tunnel: w76 -> [w103 _]
          tunnel: w75 -> [w102 _]
          tunnel: w73 -> [w101 _]
          tunnel: w72 -> [w100 _]
          frame No Error {
            n20 = flat-sequence {
              tunnel: [w129] -> w113
              tunnel: [w128] -> w112
              tunnel: w117 -> [w127]
              tunnel: w116 -> [w126]
              tunnel: w114 -> [w125]
              tunnel: [w124] -> w111
              tunnel: w110 -> [w123]
              tunnel: [w121] -> w109
              tunnel: w108 -> [w121]
              tunnel: w104 -> [w122]
              tunnel: w101 -> [w120]
              tunnel: [w194] -> w119
              tunnel: w113 -> [w193]
              tunnel: [w197] -> w118
              tunnel: w112 -> [w196]
              tunnel: [w192] -> w115
              tunnel: w111 -> [w195]
              tunnel: w109 -> [w191]
              tunnel: w107 -> [w190]
              tunnel: w106 -> [w189]
              tunnel: w105 -> [w188]
              tunnel: w103 -> [w187]
              tunnel: w102 -> [w186]
              tunnel: w100 -> [w185]
              frame #0 {
                n21 = case shown="1" w126 {
                  selector: w126 -> [w130 w144 w177]
                  tunnel: w125 -> [w132 w146 w184]
                  tunnel: [w132 w145 w183] -> w128
                  tunnel: [w131 w143 w176] -> w129
                  tunnel: w127 -> [w131 w147 w176]
                  tunnel: [w130 w144 w177] -> w124
                  tunnel: w123 -> [_ w142 _]
                  tunnel: w122 -> [_ w140 _]
                  tunnel: w120 -> [_ w135 _]
                  frame 0, Default {
                  }
                  frame 1 {
                    # "Action for command 01h: implement the received setpoints on the power supplies"
                    n22 = disable-structure shown="DEBUG==TRUE" {
                      disable-tunnel: w147 -> [w155 _]
                      disable-tunnel: w146 -> [w154 w159]
                      disable-tunnel: [w153 _] -> w143
                      disable-tunnel: [w149 w163] -> w136
                      disable-tunnel: [w148 w157] -> w134
                      frame condition #0 (active) {
                        n23 = call "LNLS Control Receive Command Body.vi"("error in (no error)"=w154, "connection ID"=w155) -> ("error out"=w150:errorcluster, "command body"=w151:string, "connection ID out"=w153:refnum<k5>)  [unwired: 6 in, 1 out]
                        n24 = call "Misc Ignore Timeout Error.vi"("error in (no error)"=w150) -> ("error out"=w152:errorcluster)  [unwired: 9 in, 1 out]
                        n25 = call "LNLS Control Decode LOCON_BIPOLAR_16BITS.vi"("error in (no error)"=w152, "command body"=w151) -> ("error out"=w148:errorcluster, "LOCON data"=w149:T19[])  [unwired: 6 in]
                      }
                      frame condition #1 {
                        n26 = flat-sequence {
                          tunnel: w159 -> [w164]
                          tunnel: [w164] -> w156
                          tunnel: ["PS Setpoints"] -> w162
                          tunnel: ["PS Status (ON/OFF)"] -> w161
                          tunnel: ["PS Status (On correction?)"] -> w160
                          tunnel: [w167] -> w158
                          tunnel: w156 -> [w167]
                          frame #0 {
                            n27 = while {
                              stop <- "send" stop-if-true
                              n28 = Wait (ms)(milliseconds to wait=u32 100) -> ()  [unwired: 1 out]
                            }
                          }
                          frame #1 {
                          }
                        }
                        n29 = call "LNLS Control PS Data to LOCON_BIPOLAR_16BITS Data.vi"("error in (no error)"=w158, "PS Status (On correction?)"=w160, "PS Status (ON/OFF)"=w161, "PS Readings/Setpoints"=w162) -> ("error out"=w157:errorcluster, "PS Readings/Setpoints LOCON Data"=w163:T19[])  [unwired: 6 in]
                      }
                    }
                    n30 = for {
                      tunnel: w136 -> [w175] mode=indexing
                      tunnel: [w173] -> w133 mode=indexing
                      n31 = Unbundle By Name(w175) -> ("status"=w172:u8)
                      n32 = Number To Boolean Array(number=w172) -> (Boolean array=w171:bool[])
                      n33 = Index Array(array=w171, index=2) -> (element=w173:bool)
                    }
                    n34 = Send Notification(notification=w133, notifier=w135) -> ()  [unwired: 1 in, 2 out]
                    n35 = call "LNLS Control LOCON_BIPOLAR_16BITS Data to PS Data.vi"("error in (no error)"=w134, "PS Setpoints LOCON Data"=w136) -> ("error out"=w145:errorcluster, "PS Status"=w141:bool[], "PS Setpoints"=w139:dbl[])  [unwired: 7 in]
                    n36 = call "Common PS Boolean to UINT8.vi"("PS ON-OFF"=w141, "Inverse PS Matrix Mapping"=w142) -> ("PS ON-OFF (per PS Rack)"=w138:u8[])  [unwired: 8 in, 1 out]
                    n37 = Build Array (concatenate)(w139, w138) -> (w137:dbl[])
                    n38 = RT FIFO Write(0:w140, 1:w137) -> ()  [unwired: 3 in, 4 out]
                  }
                  frame 4 {
                    w182 = 1 items=["Configuration Mode"=1, "Active Mode"=2] ("mode (Active Mode)")
                    # "Action for command 04h: reboot EtherCAT masters"
                    n39 = call <vilib>:"Get Scan Engine Mode.vi"("error in (no error)"=w184) -> ("error out"=w181:errorcluster, "mode"=w178:i32)  [unwired: 9 in]
                    n40 = call <vilib>:"Set Scan Engine Mode.vi"("mode (Active Mode)"=w182, "error in (no error)"=w181) -> ("error out"=w180:errorcluster)  [unwired: 13 in]
                    n41 = call <vilib>:"Clear All Faults.vi"("error in (no error)"=w180) -> ("error out"=w179:errorcluster)  [unwired: 1 in, 9 out]
                    n42 = call <vilib>:"Set Scan Engine Mode.vi"("mode (Active Mode)"=w178, "error in (no error)"=w179) -> ("error out"=w183:errorcluster)  [unwired: 13 in]
                  }
                }
              }
              frame #1 {
                n43 = case shown="0, Default" w195 {
                  tunnel: w196 -> [w213 w236]
                  tunnel: [w214 w239] -> w197
                  tunnel: [w218 w238] -> w194
                  tunnel: w193 -> [w218 w238]
                  tunnel: [w215 w237] -> w192
                  tunnel: w191 -> [w212 w235]
                  tunnel: w190 -> [_ w226]
                  tunnel: w189 -> [w198 _]
                  tunnel: w188 -> [w210 _]
                  tunnel: w187 -> [_ w234]
                  tunnel: w186 -> [w207 w233]
                  tunnel: w185 -> [w199 w227]
                  frame 0, Default {
                    w216 = u8 0  # command ID
                    # "Response to command 00h and any other: send data block containing power supplies' setpoints and status"
                    n44 = call "Common PS UINT8 to Boolean.vi"("error in (no error)"=w213, "PS Matrix Mapping"=w212, "PS Status (per PS Rack)"=w210) -> ("error out"=w206:errorcluster, "PS Status"=w208:bool[])  [unwired: 7 in]
                    n45 = Wait on Notification(notifier=w207, timeout in ms (-1)=0, error in (no error)=w206) -> (notification=w203:bool[], timed out?=w204:bool, error out=w205:errorcluster)  [unwired: 1 in, 1 out]
                    n46 = feedback #1(w199) -> (w200:bool[])
                    n47 = case shown="True" w204 {
                      tunnel: w203 -> [w219 _]
                      tunnel: [w219 w220] -> w201
                      tunnel: w200 -> [_ w220]
                      frame False {
                      }
                      frame True {
                      }
                    }
                    n48 = feedback-in #1(w201) -> ()
                    n49 = call "LNLS Control PS Data to LOCON_BIPOLAR_16BITS Data.vi"("error in (no error)"=w205, "PS Status (On correction?)"=w201, "PS Status (ON/OFF)"=w208, "PS Readings/Setpoints"=w198) -> ("error out"=w217:errorcluster, "PS Readings/Setpoints LOCON Data"=w209:T19[])  [unwired: 6 in]
                    n50 = call "LNLS Control Encode LOCON_BIPOLAR_16BITS.vi"("error in (no error)"=w217, "LOCON Data"=w209) -> ("error out"=w214:errorcluster, "command body"=w211:string)  [unwired: 8 in]
                    n51 = Bundle("command ID"=w216, "command body"=w211) -> (w215:cluster{"command ID":u8, "command body":string})  [unwired: 1 in]
                  }
                  frame 9 {
                    w240 = u8 9  # command ID
                    # "Response to command 09h: send data block containing power supplies' commands used in the orbit feedback"
                    n52 = call "Common PS UINT8 to Boolean.vi"("error in (no error)"=w236, "PS Matrix Mapping"=w235, "PS Status (per PS Rack)"=w234) -> ("error out"=w232:errorcluster, "PS Status"=w225:bool[])  [unwired: 7 in]
                    n53 = Wait on Notification(notifier=w233, timeout in ms (-1)=0, error in (no error)=w232) -> (notification=w229:bool[], timed out?=w228:bool, error out=w223:errorcluster)  [unwired: 1 in, 1 out]
                    n54 = feedback #2(w227) -> (w230:bool[])
                    n55 = case shown="False" w228 {
                      tunnel: w229 -> [w242 _]
                      tunnel: [w242 w243] -> w224
                      tunnel: w230 -> [_ w243]
                      frame False {
                      }
                      frame True {
                      }
                    }
                    n56 = feedback-in #2(w224) -> ()
                    n57 = call "LNLS Control PS Data to LOCON_BIPOLAR_16BITS Data_Command9.vi"("error in (no error)"=w223, "PS Status (On correction?)"=w224, "PS Status (ON/OFF)"=w225, "PS Readings/Setpoints"=w226) -> ("error out"=w221:errorcluster, "PS Readings/Setpoints LOCON Data"=w222:T19[])  [unwired: 6 in]
                    n58 = call "LNLS Control Encode LOCON_BIPOLAR_16BITS.vi"("error in (no error)"=w221, "LOCON Data"=w222) -> ("error out"=w239:errorcluster, "command body"=w241:string)  [unwired: 8 in]
                    n59 = Bundle("command ID"=w240, "command body"=w241) -> (w237:cluster{"command ID":u8, "command body":string})  [unwired: 1 in]
                  }
                }
              }
            }
          }
          frame Error {
            n60 = call "Misc Ignore Timeout Error.vi"("error in (no error)"=w244) -> ("error out"=w245:errorcluster)  [unwired: 9 in, 1 out]
          }
        }
        n61 = Select(t=Type_TCP_State."Close Connection", s=w89, f=Type_TCP_State."Write Data") -> (s? t:f=w90:T10)
      }
      frame "Write Data" {
        n62 = Unbundle By Name(w254) -> ("command body"=w248:string, "command ID"=w249:u8)
        n63 = disable-structure shown="DEBUG==TRUE" {
          disable-tunnel: w253 -> [w264 w273]
          disable-tunnel: w252 -> [w263 w274]
          disable-tunnel: [w262 w273] -> w251
          disable-tunnel: [w261 w274] -> w250
          disable-tunnel: w249 -> [w260 _]
          disable-tunnel: w248 -> [w258 _]
          frame condition #0 (active) {
            n64 = String Length(string=w258) -> (length=w259:i32)
            n65 = case shown="1, Default" w259 {
              tunnel: w258 -> [_ w272]
              tunnel: w264 -> [w266 w271]
              tunnel: w263 -> [w265 w270]
              tunnel: [w266 w269] -> w262
              tunnel: [w265 w268] -> w261
              tunnel: w260 -> [_ w267]
              frame 0 {
              }
              frame 1, Default {
                n66 = call "LNLS Control Send Command.vi"("command body"=w272, "error in (no error)"=w270, "command ID"=w267, "connection ID"=w271) -> ("error out"=w268:errorcluster, "connection ID out"=w269:refnum<k5>)  [unwired: 6 in]
              }
            }
          }
          frame condition #1 {
          }
        }
        n67 = Select(t=Type_TCP_State."Close Connection", s=w250, f=Type_TCP_State."Read Data") -> (s? t:f=w255:T10)
      }
      frame "Close Connection" {
        n68 = disable-structure shown="DEBUG==TRUE" {
          disable-tunnel: w279 -> [w284 w285]
          disable-tunnel: [w283 w285] -> w278
          disable-tunnel: w276 -> [w282 w286]
          disable-tunnel: [w280 w286] -> w275
          frame condition #0 (active) {
            n69 = TCP Close Connection(connection ID=w284) -> (connection ID out=w283:refnum<k5>, error out=w281:errorcluster)  [unwired: 2 in]
            n70 = Merge Errors(w281, w282) -> (w280:errorcluster)
          }
          frame condition #1 {
          }
        }
      }
    }
    n71 = node-c288() -> ()  [unwired: 1 in, 1 out]
  }
  "error out" <- w18
  n72 = node-c288(w9) -> ()  [unwired: 1 out]
